vi "Thor_GetStatus.vi"(8 "error in (no error)":errorcluster, 10 "Device In":T1, 11 "KCubeServoControl In":T2) -> (0 "error out":errorcluster, 2 "Device Out":T1, 3 "KCubeServoControl out":T2, 5 "Z Moving?":bool, 7 "HW LimitSwitches":bool)   [LabVIEW 2020]
uses:
  Thor_KCubeServoDCRef.ctl
  E:/Norway Project/All Hardware/New Microscope/LabVIEW/ThorLabs/Thorlabs.MotionControl.Controls.dll
  Thorlabs.MotionControl.Controls.dll
  Thor_DeviceRef.ctl
  E:/Norway Project/All Hardware/New Microscope/LabVIEW/ThorLabs/ThorLabs.MotionControl.KCube.DCServoCLI.dll
  ThorLabs.MotionControl.KCube.DCServoCLI.dll
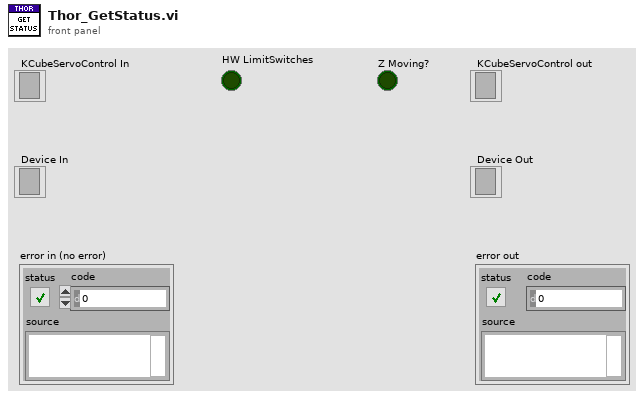
[diagram p1: front panel]
types:
  T1 = typedef "Thor_DeviceRef.ctl" = refnum<k24>
  T2 = typedef "Thor_KCubeServoDCRef.ctl" = refnum<k24>
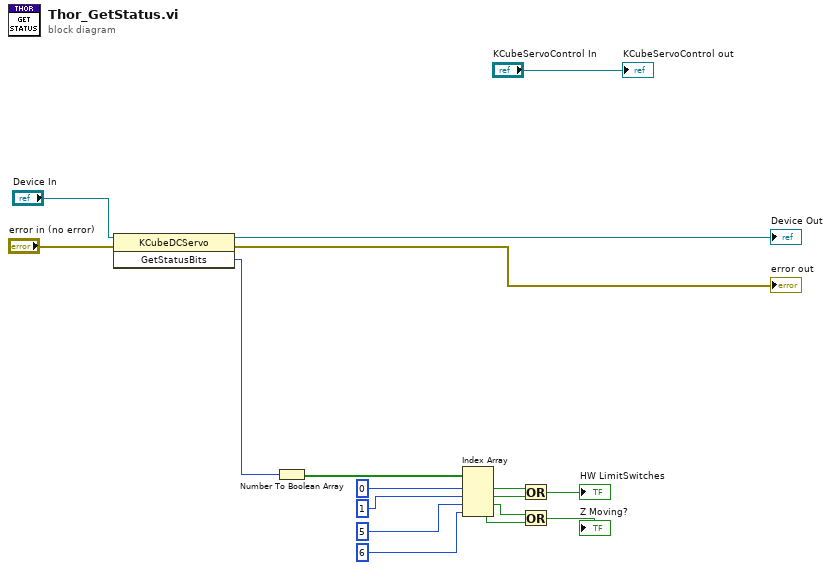
[diagram p0: block diagram]
diagram:
  n1 = invoke class="KCubeDCServo" method="GetStatusBits"(reference="Device In", error in="error in (no error)") -> (reference out=→"Device Out":T1, error out=→"error out":errorcluster, "GetStatusBits"=w12:u32)  [unwired: 1 in]
  n2 = Number To Boolean Array(number=w12) -> (Boolean array=w11:bool[])
  n3 = Index Array(array=w11, index #1=0 ("index"), index #2=1 ("index"), index #3=5 ("index"), index #4=6 ("index")) -> (element #1=w6:bool, element #2=w5:bool, element #3=w3:bool, element #4=w2:bool)
  n4 = Or(x=w6, y=w5) -> (x .or. y?=→"HW LimitSwitches":bool)
  n5 = Or(x=w3, y=w2) -> (x .or. y?=→"Z Moving?":bool)
  "KCubeServoControl out" <- "KCubeServoControl In"
